vi "CAN测试接收发送.vi"(7 "Order":u16, 8 "data_4":u16, 9 "data_3":u16, 10 "data_2":u16, 11 "data_1":u16) -> (0 "接收数据":u16[](array[numeric]), 2 "成功？":bool)   [LabVIEW 2010]
uses:
  全局量/全局_配置.vi
panel:
  in  "Send_MSG":T1(array[cluster])=[{"Flags"=4, "ID(HEX)"=0, "Data "=[0, 0, 0, 0, 0, 0, 0, 0]}, {"Flags"=4, "ID(HEX)"=0, "Data "=[0, 0, 0, 0, 0, 0, 0, 1]}, {"Flags"=4, "ID(HEX)"=0, "Data "=[0, 0, 0, 0, 0, 0, 0, 2]}, {"Flags"=4, "ID(HEX)"=0, "Data "=[0, 0, 0, 0, 0, 0, 0, 3]}, {"Flags"=4, "ID(HEX)"=0, "Data "=[0, 0, 0, 0, 0, 0, 0, 4]}, {"Flags"=4, "ID(HEX)"=0, "Data "=[0, 0, 0, 0, 0, 0, 0, 5]}, {"Flags"=4, "ID(HEX)"=0, "Data "=[0, 0, 0, 0, 0, 0, 0, 6]}, {"Flags"=4, "ID(HEX)"=0, "Data "=[0, 0, 0, 0, 0, 0, 0, 7]}, {"Flags"=4, "ID(HEX)"=0, "Data "=[0, 0, 0, 0, 0, 0, 0, 8]}, {"Flags"=4, "ID(HEX)"=0, "Data "=[0, 0, 0, 0, 0, 0, 0, 9]}, {"Flags"=4, "ID(HEX)"=0, "Data "=[0, 0, 0, 0, 0, 0, 1, 0]}, {"Flags"=4, "ID(HEX)"=0, "Data "=[0, 0, 0, 0, 0, 0, 1, 1]}, {"Flags"=4, "ID(HEX)"=0, "Data "=[0, 0, 0, 0, 0, 0, 1, 2]}, {"Flags"=4, "ID(HEX)"=0, "Data "=[0, 0, 0, 0, 0, 0, 1, 3]}, {"Flags"=4, "ID(HEX)"=0, "Data "=[0, 0, 0, 0, 0, 0, 1, 4]}, {"Flags"=4, "ID(HEX)"=0, "Data "=[0, 0, 0, 0, 0, 0, 1, 5]}, {"Flags"=4, "ID(HEX)"=0, "Data "=[0, 0, 0, 0, 0, 0, 1, 6]}, {"Flags"=4, "ID(HEX)"=0, "Data "=[0, 0, 0, 0, 0, 0, 1, 7]}, {"Flags"=4, "ID(HEX)"=0, "Data "=[0, 0, 0, 0, 0, 0, 1, 8]}, {"Flags"=4, "ID(HEX)"=0, "Data "=[0, 0, 0, 0, 0, 0, 1, 9]}, {"Flags"=4, "ID(HEX)"=0, "Data "=[0, 0, 0, 0, 0, 0, 2, 0]}, {"Flags"=4, "ID(HEX)"=0, "Data "=[0, 0, 0, 0, 0, 0, 2, 1]}, {"Flags"=4, "ID(HEX)"=0, "Data "=[0, 0, 0, 0, 0, 0, 2, 2]}, {"Flags"=4, "ID(HEX)"=0, "Data "=[0, 0, 0, 0, 0, 0, 2, 3]}, {"Flags"=4, "ID(HEX)"=0, "Data "=[0, 0, 0, 0, 0, 0, 2, 4]}, {"Flags"=4, "ID(HEX)"=0, "Data "=[0, 0, 0, 0, 0, 0, 2, 5]}, {"Flags"=4, "ID(HEX)"=0, "Data "=[0, 0, 0, 0, 0, 0, 2, 6]}, {"Flags"=4, "ID(HEX)"=0, "Data "=[0, 0, 0, 0, 0, 0, 2, 7]}, {"Flags"=4, "ID(HEX)"=0, "Data "=[0, 0, 0, 0, 0, 0, 2, 8]}, {"Flags"=4, "ID(HEX)"=0, "Data "=[0, 0, 0, 0, 0, 0, 2, 9]}, {"Flags"=4, "ID(HEX)"=0, "Data "=[0, 0, 0, 0, 0, 0, 3, 0]}, {"Flags"=4, "ID(HEX)"=0, "Data "=[0, 0, 0, 0, 0, 0, 3, 1]}, {"Flags"=4, "ID(HEX)"=0, "Data "=[0, 0, 0, 0, 0, 0, 3, 2]}, {"Flags"=4, "ID(HEX)"=0, "Data "=[0, 0, 0, 0, 0, 0, 3, 3]}, {"Flags"=4, "ID(HEX)"=0, "Data "=[0, 0, 0, 0, 0, 0, 3, 4]}, {"Flags"=4, "ID(HEX)"=0, "Data "=[0, 0, 0, 0, 0, 0, 3, 5]}, {"Flags"=4, "ID(HEX)"=0, "Data "=[0, 0, 0, 0, 0, 0, 3, 6]}, {"Flags"=4, "ID(HEX)"=0, "Data "=[0, 0, 0, 0, 0, 0, 3, 7]}, {"Flags"=4, "ID(HEX)"=0, "Data "=[0, 0, 0, 0, 0, 0, 3, 8]}, {"Flags"=4, "ID(HEX)"=0, "Data "=[0, 0, 0, 0, 0, 0, 3, 9]}, {"Flags"=4, "ID(HEX)"=0, "Data "=[0, 0, 0, 0, 0, 0, 4, 0]}, {"Flags"=4, "ID(HEX)"=0, "Data "=[0, 0, 0, 0, 0, 0, 4, 1]}, {"Flags"=4, "ID(HEX)"=0, "Data "=[0, 0, 0, 0, 0, 0, 4, 2]}, {"Flags"=4, "ID(HEX)"=0, "Data "=[0, 0, 0, 0, 0, 0, 4, 3]}, {"Flags"=4, "ID(HEX)"=0, "Data "=[0, 0, 0, 0, 0, 0, 4, 4]}, {"Flags"=4, "ID(HEX)"=0, "Data "=[0, 0, 0, 0, 0, 0, 4, 5]}, {"Flags"=4, "ID(HEX)"=0, "Data "=[0, 0, 0, 0, 0, 0, 4, 6]}, {"Flags"=4, "ID(HEX)"=0, "Data "=[0, 0, 0, 0, 0, 0, 4, 7]}, {"Flags"=4, "ID(HEX)"=0, "Data "=[0, 0, 0, 0, 0, 0, 4, 8]}, {"Flags"=4, "ID(HEX)"=0, "Data "=[0, 0, 0, 0, 0, 0, 4, 9]}, {"Flags"=4, "ID(HEX)"=0, "Data "=[0, 0, 0, 0, 0, 0, 5, 0]}, {"Flags"=4, "ID(HEX)"=0, "Data "=[0, 0, 0, 0, 0, 0, 5, 1]}, {"Flags"=4, "ID(HEX)"=0, "Data "=[0, 0, 0, 0, 0, 0, 5, 2]}, {"Flags"=4, "ID(HEX)"=0, "Data "=[0, 0, 0, 0, 0, 0, 5, 3]}, {"Flags"=4, "ID(HEX)"=0, "Data "=[0, 0, 0, 0, 0, 0, 5, 4]}, {"Flags"=4, "ID(HEX)"=0, "Data "=[0, 0, 0, 0, 0, 0, 5, 5]}, {"Flags"=4, "ID(HEX)"=0, "Data "=[0, 0, 0, 0, 0, 0, 5, 6]}, {"Flags"=4, "ID(HEX)"=0, "Data "=[0, 0, 0, 0, 0, 0, 5, 7]}, {"Flags"=4, "ID(HEX)"=0, "Data "=[0, 0, 0, 0, 0, 0, 5, 8]}, {"Flags"=4, "ID(HEX)"=0, "Data "=[0, 0, 0, 0, 0, 0, 5, 9]}, {"Flags"=4, "ID(HEX)"=0, "Data "=[0, 0, 0, 0, 0, 0, 6, 0]}, {"Flags"=4, "ID(HEX)"=0, "Data "=[0, 0, 0, 0, 0, 0, 6, 1]}, {"Flags"=4, "ID(HEX)"=0, "Data "=[0, 0, 0, 0, 0, 0, 6, 2]}, {"Flags"=4, "ID(HEX)"=0, "Data "=[0, 0, 0, 0, 0, 0, 6, 3]}, {"Flags"=4, "ID(HEX)"=0, "Data "=[0, 0, 0, 0, 0, 0, 6, 4]}, {"Flags"=4, "ID(HEX)"=0, "Data "=[0, 0, 0, 0, 0, 0, 6, 5]}, {"Flags"=4, "ID(HEX)"=0, "Data "=[0, 0, 0, 0, 0, 0, 6, 6]}, {"Flags"=4, "ID(HEX)"=0, "Data "=[0, 0, 0, 0, 0, 0, 6, 7]}, {"Flags"=4, "ID(HEX)"=0, "Data "=[0, 0, 0, 0, 0, 0, 6, 8]}, {"Flags"=4, "ID(HEX)"=0, "Data "=[0, 0, 0, 0, 0, 0, 6, 9]}, {"Flags"=4, "ID(HEX)"=0, "Data "=[0, 0, 0, 0, 0, 0, 7, 0]}, {"Flags"=4, "ID(HEX)"=0, "Data "=[0, 0, 0, 0, 0, 0, 7, 1]}, {"Flags"=4, "ID(HEX)"=0, "Data "=[0, 0, 0, 0, 0, 0, 7, 2]}, {"Flags"=4, "ID(HEX)"=0, "Data "=[0, 0, 0, 0, 0, 0, 7, 3]}, {"Flags"=4, "ID(HEX)"=0, "Data "=[0, 0, 0, 0, 0, 0, 7, 4]}, {"Flags"=4, "ID(HEX)"=0, "Data "=[0, 0, 0, 0, 0, 0, 7, 5]}, {"Flags"=4, "ID(HEX)"=0, "Data "=[0, 0, 0, 0, 0, 0, 7, 6]}, {"Flags"=4, "ID(HEX)"=0, "Data "=[0, 0, 0, 0, 0, 0, 7, 7]}, {"Flags"=4, "ID(HEX)"=0, "Data "=[0, 0, 0, 0, 0, 0, 7, 8]}, {"Flags"=4, "ID(HEX)"=0, "Data "=[0, 0, 0, 0, 0, 0, 7, 9]}, {"Flags"=4, "ID(HEX)"=0, "Data "=[0, 0, 0, 0, 0, 0, 8, 0]}, {"Flags"=4, "ID(HEX)"=0, "Data "=[0, 0, 0, 0, 0, 0, 8, 1]}, {"Flags"=4, "ID(HEX)"=0, "Data "=[0, 0, 0, 0, 0, 0, 8, 2]}, {"Flags"=4, "ID(HEX)"=0, "Data "=[0, 0, 0, 0, 0, 0, 8, 3]}, {"Flags"=4, "ID(HEX)"=0, "Data "=[0, 0, 0, 0, 0, 0, 8, 4]}, {"Flags"=4, "ID(HEX)"=0, "Data "=[0, 0, 0, 0, 0, 0, 8, 5]}, {"Flags"=4, "ID(HEX)"=0, "Data "=[0, 0, 0, 0, 0, 0, 8, 6]}, {"Flags"=4, "ID(HEX)"=0, "Data "=[0, 0, 0, 0, 0, 0, 8, 7]}, {"Flags"=4, "ID(HEX)"=0, "Data "=[0, 0, 0, 0, 0, 0, 8, 8]}, {"Flags"=4, "ID(HEX)"=0, "Data "=[0, 0, 0, 0, 0, 0, 8, 9]}, {"Flags"=4, "ID(HEX)"=0, "Data "=[0, 0, 0, 0, 0, 0, 9, 0]}, {"Flags"=4, "ID(HEX)"=0, "Data "=[0, 0, 0, 0, 0, 0, 9, 1]}, {"Flags"=4, "ID(HEX)"=0, "Data "=[0, 0, 0, 0, 0, 0, 9, 2]}, {"Flags"=4, "ID(HEX)"=0, "Data "=[0, 0, 0, 0, 0, 0, 9, 3]}, {"Flags"=4, "ID(HEX)"=0, "Data "=[0, 0, 0, 0, 0, 0, 9, 4]}, {"Flags"=4, "ID(HEX)"=0, "Data "=[0, 0, 0, 0, 0, 0, 9, 5]}, {"Flags"=4, "ID(HEX)"=0, "Data "=[0, 0, 0, 0, 0, 0, 9, 6]}, {"Flags"=4, "ID(HEX)"=0, "Data "=[0, 0, 0, 0, 0, 0, 9, 7]}, {"Flags"=4, "ID(HEX)"=0, "Data "=[0, 0, 0, 0, 0, 0, 9, 8]}, {"Flags"=4, "ID(HEX)"=0, "Data "=[0, 0, 0, 0, 0, 0, 9, 9]}] {"Data" format="%x"; "Flags" items=["MSG_STD"=0, "MSG_EXT"=4]; "ID(HEX)" format="%x"}
  out "开始时间":dbl format="%#.0f"
  out "Error out":errorcluster {"code" format="%.0x"}
  in  "ReadTimeOut":u32=3000 caption="ms"
  in  "Synchronization":i32(ring)=1 items=["Synchronization"=1, "Asynchronization"=0]
  # "从0开始"
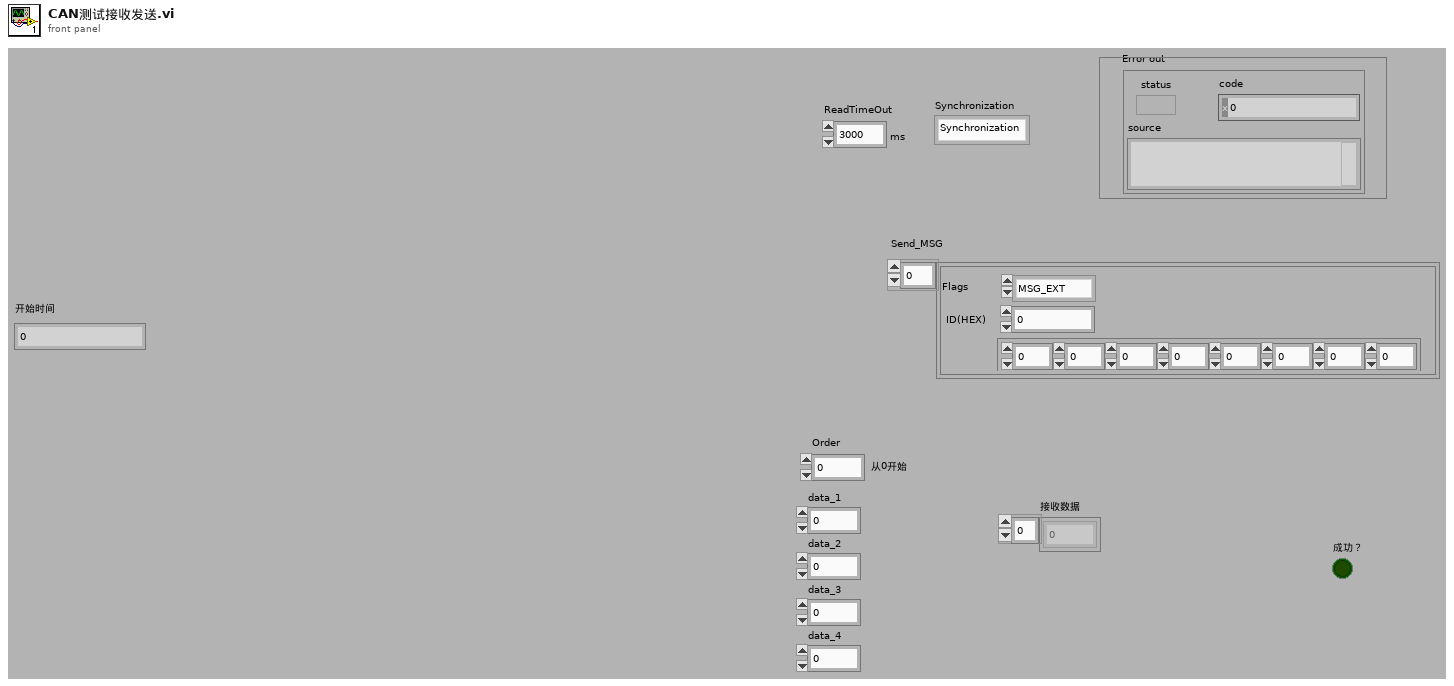
[diagram p1: front panel]
types:
  T1 = cluster{"Flags":u32, "ID(HEX)":u32, "Data ":u8[]}[]
  T2 = cluster{"Internal":u32, "InternalHigh":u32, "Offset":u32, "OffsetHigh":u32, "hEvent":u32}
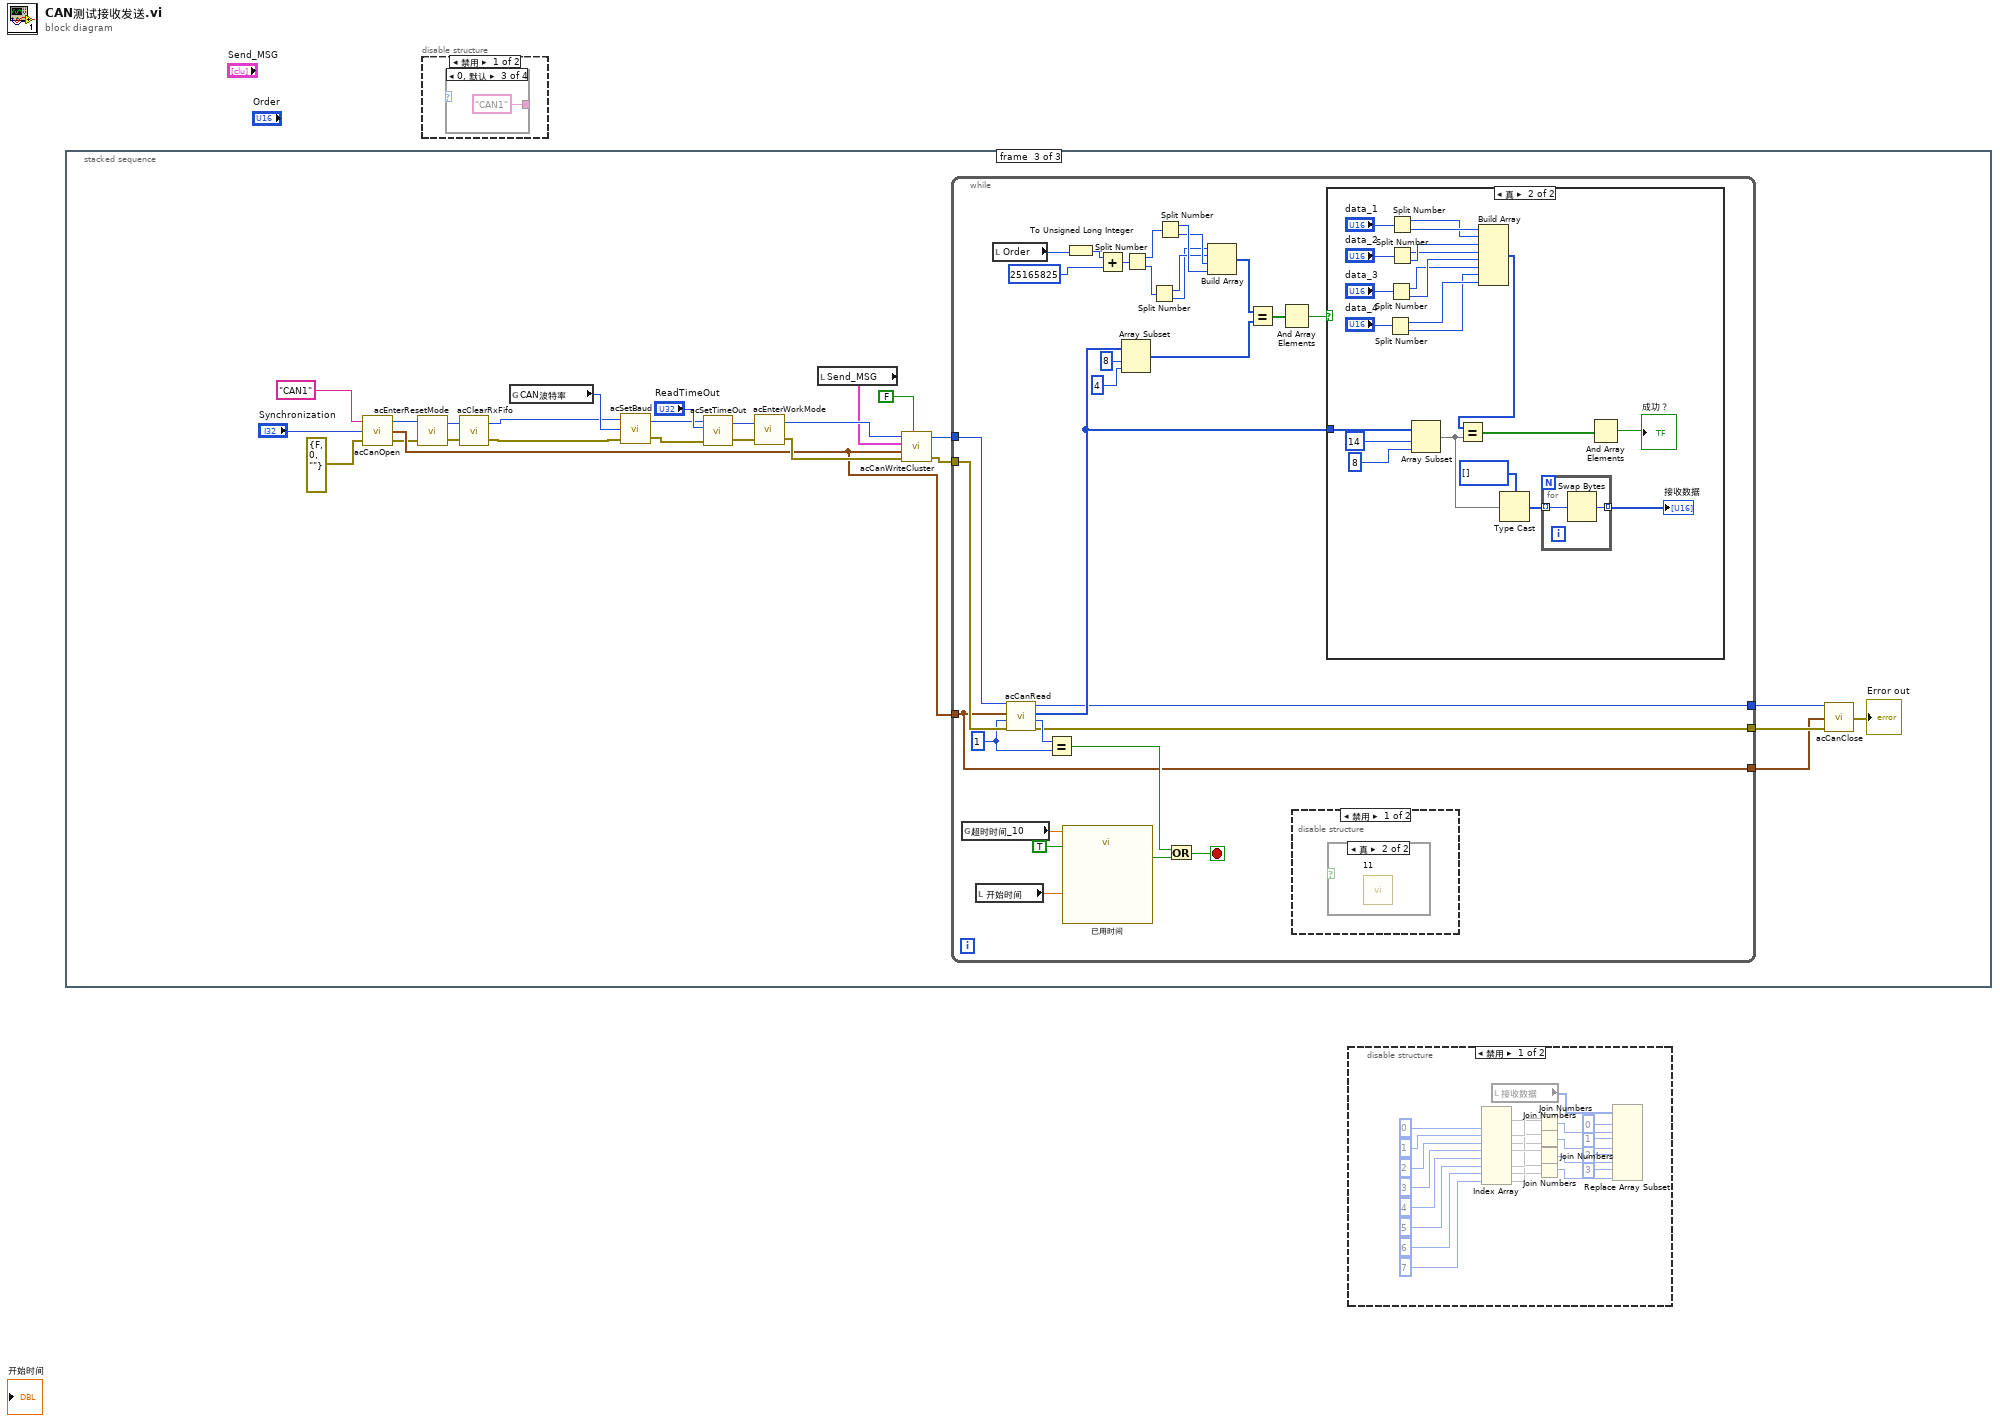
[diagram p0: block diagram]
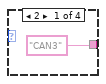
[diagram p2: hidden frame]
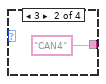
[diagram p3: hidden frame]
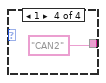
[diagram p4: hidden frame]
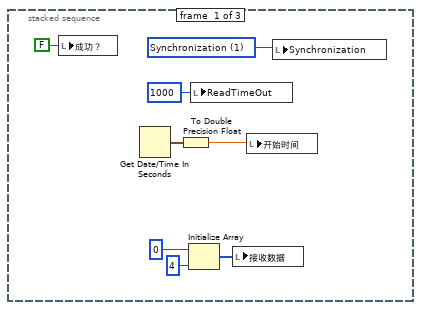
[diagram p7: hidden frame]
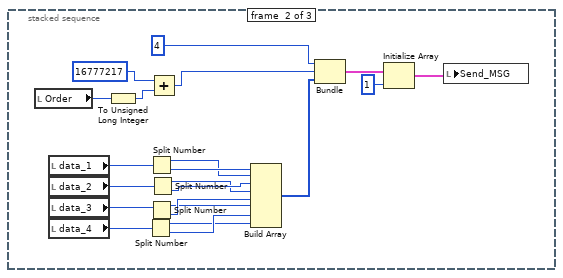
[diagram p8: hidden frame]
diagram:
  n1 = stacked-sequence {
    frame #0 {
      w6 = 1 items=["Synchronization"=1, "Asynchronization"=0] ("Synchronization")
      n2 = local write "成功？"(FALSE ("成功？")) -> ()
      n3 = Get Date/Time In Seconds() -> (seconds since 1Jan1904=w2:timestamp)
      n4 = To Double Precision Float(number=w2) -> (double precision float=w1:dbl)
      n5 = Initialize Array(u16 0, 4 ("维数大小")) -> (w3:u16[])
      n6 = local write "ReadTimeOut"(u32 1000 ("ReadTimeOut")) -> ()
      n7 = local write "接收数据"(w3) -> ()
      n8 = local write "开始时间"(w1) -> ()
      n9 = local write "Synchronization"(w6) -> ()
    }
    frame #1 {
      n10 = local read "Order"() -> (w10:u16)
      n11 = local read "data_1"() -> (w14:u16)
      n12 = local read "data_2"() -> (w13:u16)
      n13 = local read "data_3"() -> (w12:u16)
      n14 = local read "data_4"() -> (w11:u16)
      n15 = To Unsigned Long Integer(number=w10) -> (unsigned 32bit integer=w29:u32)
      n16 = Split Number(x=w11) -> (hi(x)=w24:u8, lo(x)=w25:u8)
      n17 = Split Number(x=w14) -> (hi(x)=w18:u8, lo(x)=w19:u8)
      n18 = Split Number(x=w12) -> (hi(x)=w22:u8, lo(x)=w23:u8)
      n19 = Split Number(x=w13) -> (hi(x)=w20:u8, lo(x)=w21:u8)
      n20 = Add(x=u32 16777217, y=w29) -> (x+y=w28:u32)
      n21 = Build Array(w19, w18, w21, w20, w23, w22, w25, w24) -> (w17:u8[])
      n22 = Bundle(u32 4, w28, w17) -> (w15:cluster{u32, u32, u8[]})  [unwired: 1 in]
      n23 = Initialize Array(w15, 1 ("维数大小")) -> (w9:cluster{u32, u32, u8[]}[])
      n24 = local write "Send_MSG"(w9) -> ()
    }
    frame #2 {
      n25 = call "acCanOpen.vi"("Error in"=errorcluster {"status"=FALSE, "code"=0, "source"=""}, "Synchronization"="Synchronization", "CANPort"="CAN1") -> ("Error out"=w32:errorcluster, "Overlapped"=w49:T2, "Handle"=w31:u32)
      n26 = call "acEnterResetMode.vi"("Error in"=w32, "Handle  in"=w31) -> ("Error out"=w38:errorcluster, "Handle out"=w39:u32)
      n27 = call "acClearRxFifo.vi"("Error in"=w38, "Handle  in"=w39) -> ("Error out"=w41:errorcluster, "Handle out"=w40:u32)
      n28 = global read "全局_配置.vi" "CAN波特率"() -> (w44:u16)
      n29 = call "acSetBaud.vi"("Error in"=w41, "Baudrate"=w44, "Handle  in"=w40) -> ("Error out"=w36:errorcluster, "Handle out"=w35:u32)
      n30 = call "acSetTimeOut.vi"("Error in"=w36, "Read TimeOut"="ReadTimeOut", "Handle  in"=w35) -> ("Error out"=w43:errorcluster, "Handle out"=w42:u32)  [unwired: 1 in]
      n31 = call "acEnterWorkMode.vi"("Error in"=w43, "Handle  in"=w42) -> ("Error out"=w52:errorcluster, "Handle out"=w55:u32)
      n32 = local read "Send_MSG"() -> (w53:T1)
      n33 = call "acCanWriteCluster.vi"("Handle  in"=w55, "MSG"=w53, "Overlapped"=w49, "Error in"=w52, "MSG_RTR"=FALSE) -> ("Handle out"=w50:u32, "Error out"=w51:errorcluster)  [unwired: 1 out]
      n34 = while {
        tunnel: w51 -> [w66]
        tunnel: w50 -> [w67]
        tunnel: w49 -> [w57]
        tunnel: [w59] -> w47
        tunnel: [w58] -> w46
        tunnel: [w57] -> w45
        stop <- w60 stop-if-true
        w61 = u32 1 ("ReadCount")
        n35 = global read "全局_配置.vi" "超时时间_10"() -> (w64:dbl)
        n36 = local read "开始时间"() -> (w63:dbl)
        n37 = local read "Order"() -> (w84:u16)
        n38 = call "acCanRead.vi"("Error in"=w66, "ReadCount"=w61, "Overlapped"=w57, "Handle  in"=w67) -> ("Error out"=w58:errorcluster, "NumberOfRead"=w85:u32, "MSG"=w68:u8[], "Handle out"=w59:u32)
        n39 = Equal?(x=w85, y=w61) -> (x = y?=w62:bool)
        n40 = call "已用时间"("Time Target (s)"=w64, "Reset"=TRUE, "Set Start Time (s)"=w63) -> ("Time has Elapsed"=w56:bool)  [unwired: 9 in, 7 out]
        n41 = To Unsigned Long Integer(number=w84) -> (unsigned 32bit integer=w70:u32)
        n42 = Add(x=w70, y=u32 25165825) -> (x+y=w71:u32)
        n43 = Array Subset(array=w68, index=8 ("索引"), length=4 ("长度")) -> (w81:u8[])
        n44 = Split Number(x=w71) -> (hi(x)=w72:u16, lo(x)=w73:u16)
        n45 = Split Number(x=w73) -> (hi(x)=w75:u8, lo(x)=w74:u8)
        n46 = Split Number(x=w72) -> (hi(x)=w77:u8, lo(x)=w76:u8)
        n47 = Or(x=w62, y=w56) -> (x .or. y?=w60:bool)
        n48 = Build Array(w74, w75, w76, w77) -> (w80:u8[])
        n49 = Equal?(x=w80, y=w81) -> (x = y?=w82:bool[])
        n50 = And Array Elements(Boolean array=w82) -> (logical AND=w83:bool)
        n51 = disable-structure shown="禁用" {
          frame Disabled {
            n52 = case shown="真" {
              selector: _ -> [_ _]
              frame False {
              }
              frame True {
                n53 = call "11"() -> ()  [unwired: 10 in, 2 out]
              }
            }
          }
          frame Enabled {
          }
        }
        n54 = case shown="真" w83 {
          tunnel: w68 -> [_ w90]
          frame False {
          }
          frame True {
            n55 = Split Number(x="data_4") -> (hi(x)=w96:u8, lo(x)=w95:u8)
            n56 = Split Number(x="data_3") -> (hi(x)=w97:u8, lo(x)=w98:u8)
            n57 = Split Number(x="data_1") -> (hi(x)=w101:u8, lo(x)=w102:u8)
            n58 = Split Number(x="data_2") -> (hi(x)=w99:u8, lo(x)=w100:u8)
            n59 = Array Subset(array=w90, index=14 ("索引"), length=8 ("长度")) -> (w89:u8[])
            n60 = Build Array(w102, w101, w100, w99, w98, w97, w95, w96) -> (w91:u8[])
            n61 = Equal?(x=w91, y=w89) -> (x = y?=w107:bool[])
            n62 = Type Cast(type=u16[] [], x=w89) -> (*(type *) &x=w87:u16[])
            n63 = for {
              tunnel: w87 -> [w109] mode=indexing
              tunnel: [w108] -> w86 mode=indexing
              n64 = Swap Bytes(anything=w109) -> (byte swapped=w108:u16)
            }
            "接收数据" <- w86
            n65 = And Array Elements ("数组元素与操作")(Boolean array=w107) -> (logical AND=→"成功？":bool)
          }
        }
      }
      n66 = call "acCanClose.vi"("Error in"=w46, "Overlapped"=w45, "Handle  in"=w47) -> ("Error out"=→"Error out":errorcluster)
    }
  }
  n67 = disable-structure shown="禁用" {
    frame Disabled {
      n68 = case shown="0, 默认" {
        selector: _ -> [_ _ _ _]
        tunnel: ["CAN3" "CAN4" "CAN1" "CAN2"] -> _
        frame 2 {
        }
        frame 3 {
        }
        frame 0, Default {
        }
        frame 1 {
        }
      }
    }
    frame Enabled {
    }
  }
  n69 = disable-structure shown="禁用" {
    frame Disabled {
      n70 = Index Array(index #1=0 ("索引"), index #2=1 ("索引"), index #3=2 ("索引"), index #4=3 ("索引"), index #5=4 ("索引"), index #6=5 ("索引"), index #7=6 ("索引"), index #8=7 ("索引")) -> (array=w114:u8[], element #1=w130, element #2=w131, element #3=w128, element #4=w129, element #5=w127, element #6=w126, element #7=w116, element #8=w115)
      n71 = local read "接收数据"() -> (w125:u16[])
      n72 = Join Numbers(hi=w131, lo=w130) -> ((hi.lo)=w123:u32)
      n73 = Join Numbers(hi=w129, lo=w128) -> ((hi.lo)=w121:u32)
      n74 = Join Numbers(hi=w126, lo=w127) -> ((hi.lo)=w119:u32)
      n75 = Join Numbers(hi=w116, lo=w115) -> ((hi.lo)=w117:u32)
      n76 = Replace Array Subset(array=w125, new element #1=w123, index #1=0 ("索引"), new element #2=w121, index #2=1 ("索引"), new element #3=w119, index #3=2 ("索引"), new element #4=w117, index #4=3 ("索引")) -> ()  [unwired: 1 out]
    }
    frame Enabled {
    }
  }
